vi "dashboard.vi"() -> ()   [LabVIEW 2022 SP3]
panel:
  in  "Stop":bool
  out "Write Count":i32
  out "Read Count":i32
  in  "Reset Communication":bool
  in  "USB Port":refnum<visa-resource-name>
  out "u":dbl format="%.2g"
  out "D":dbl format="%.2g"
  out "I":dbl format="%.2g"
  out "P":dbl format="%.2g"
  in  "Tau D (s)":dbl=11.370000000000003 min=0.0 max=30.0 step=0.01 format="%.2g"
  in  "Kd":dbl=46.0 min=0.0 max=50.0 step=0.01 format="%.2g"
  in  "Ki":dbl=49.920000000000016 min=0.0 max=50.0 step=0.01 format="%.2g"
  in  "Kp":dbl=37.15999999999997 min=0.0 max=50.0 step=0.01 format="%.2g"
  in  "Motor Enable":bool
  in  "Speed Reference (RPM)":dbl=100.0 min=0.0 max=1500.0 step=50.0 format="%#.3g"
  out "Flag AntiWindUp":bool
  in  "Tau Error (s)":dbl=8.649999999999995 min=0.0 max=30.0 step=0.01 format="%.2g"
  out "Filtered Error (°)":dbl
  out "Error (°)":dbl
  out "Controller":cluster{" P":dbl, "I":dbl, "D":dbl, "u":dbl}(graph)
  out "Error":cluster{" error":dbl, "Filtered_error":dbl}(graph)
  out "IR Sensors":bool[](array[boolean])
  in  "Right Motor Speed (RPM)":dbl(slide) min=-1500.0 max=1500.0 step=100.0 scale=-1500.0..1500.0
  in  "Left Motor Speed (RPM)":dbl(slide) min=-1500.0 max=1500.0 step=100.0 scale=-1500.0..1500.0
  in  "Manual Control":bool
  out "Left Motor":cluster{"l_sp":dbl, "l_speed":dbl}(graph)
  out "Right Motor":cluster{"r_sp":dbl, " r_speed":dbl}(graph)
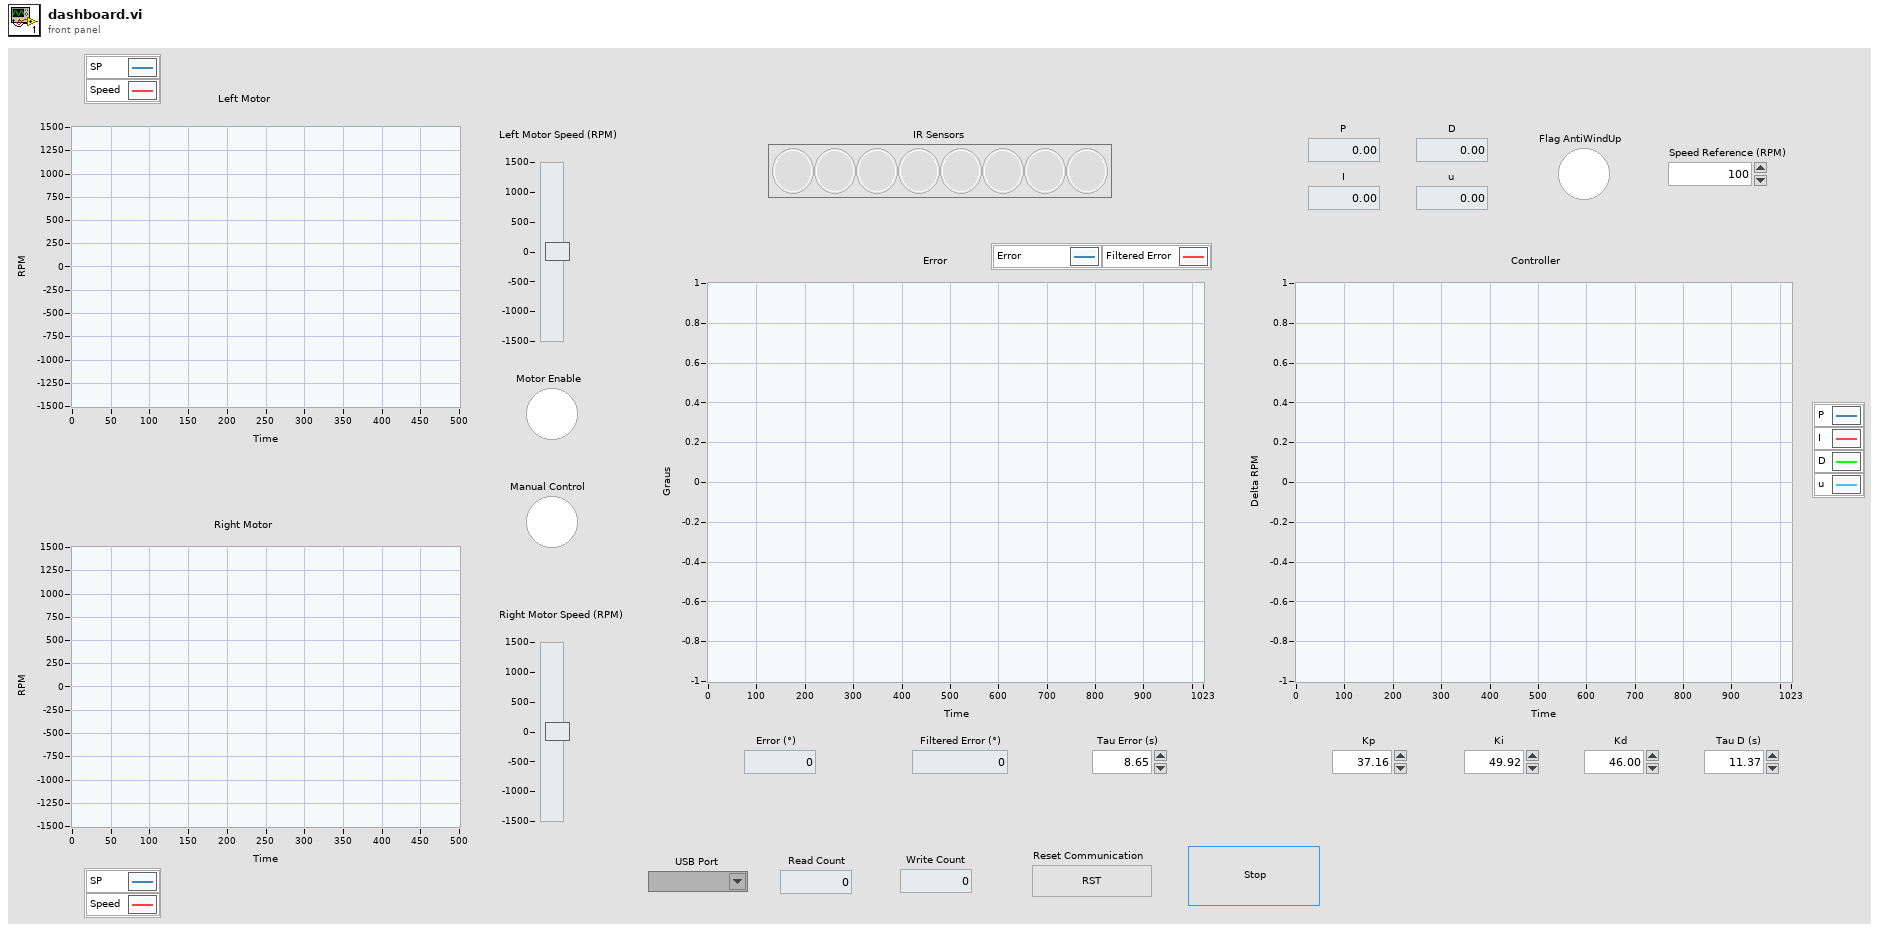
[diagram p1: front panel]
types:
  T1 = cluster{"Manual Control":bool, "Motor Enable":bool, "Left Motor Speed (RPM)":dbl, "Right Motor Speed (RPM)":dbl, "Tau Error (s)":dbl, "Kp":dbl, "Ki":dbl, "Kd":dbl, "Tau D (s)":dbl, "Speed Reference (RPM)":dbl, dbl, dbl, dbl, dbl, dbl, dbl}
  T2 = cluster{"l_sp":dbl, "l_speed":dbl, "r_sp":dbl, " r_speed":dbl, " error":dbl, "Filtered_error":dbl, " P":dbl, "I":dbl, "D":dbl, "u":dbl, "sat_flag":bool, " IR":bool[], "A_":dbl, " B_":dbl, " C_":dbl, "D_":dbl}
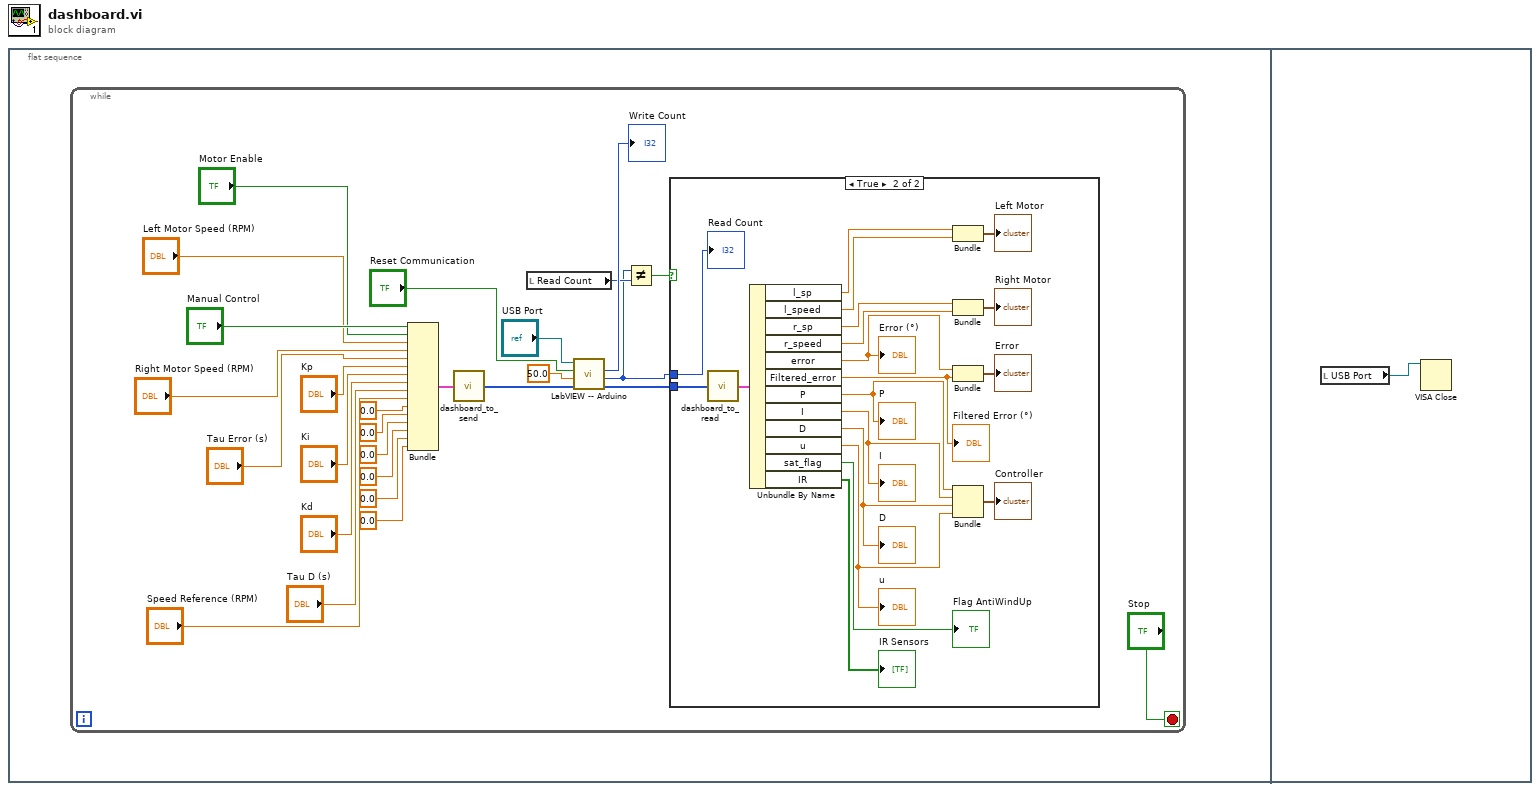
[diagram p0: block diagram]
diagram:
  n1 = flat-sequence {
    frame #0 {
      n2 = while {
        stop <- "Stop" stop-if-true
        n3 = Bundle("Manual Control"="Manual Control", "Motor Enable"="Motor Enable", "Left Motor Speed (RPM)"="Left Motor Speed (RPM)", "Right Motor Speed (RPM)"="Right Motor Speed (RPM)", "Tau Error (s)"="Tau Error (s)", "Kp"="Kp", "Ki"="Ki", "Kd"="Kd", "Tau D (s)"="Tau D (s)", "Speed Reference (RPM)"="Speed Reference (RPM)", 0.0, 0.0, 0.0, 0.0, 0.0, 0.0) -> (w6:T1)  [unwired: 1 in]
        n4 = call "dashboard_to_send.vi"("In"=w6) -> ("Output"=w5:u8[])
        n5 = local read "Read Count"() -> (w3:i32)
        n6 = call "LabVIEW -- Arduino.vi"("Data to Write"=w5, "Frequency Write"=50.0, "Reset"="Reset Communication", "VISA resource name"="USB Port") -> ("Read Data"=w1:u8[], "Read Count"=w2:i32, "Write Count"=→"Write Count":u16)  [unwired: 1 out]
        n7 = Not Equal?(x=w2, y=w3) -> (x != y?=w4:bool)
        n8 = case shown="True" w4 {
          tunnel: w2 -> [_ w46]
          tunnel: w1 -> [_ w45]
          frame False {
          }
          frame True {
            n9 = call "dashboard_to_read.vi"("In"=w45) -> ("Out"=w44:T2)
            n10 = Unbundle By Name(w44) -> ("l_sp"=w42:dbl, "l_speed"=w41:dbl, "r_sp"=w39:dbl, "r_speed"=w38:dbl, "error"=w33:dbl, "Filtered_error"=w32:dbl, "P"=w31:dbl, "I"=w30:dbl, "D"=w29:dbl, "u"=w28:dbl, "sat_flag"=→"Flag AntiWindUp":bool, "IR"=→"IR Sensors":bool[])
            "Error (°)" <- w33
            "Filtered Error (°)" <- w32
            "P" <- w31
            "I" <- w30
            "D" <- w29
            "u" <- w28
            n11 = Bundle("l_sp"=w42, "l_speed"=w41) -> (→"Left Motor":cluster{"l_sp":dbl, "l_speed":dbl})  [unwired: 1 in]
            n12 = Bundle("r_sp"=w39, "r_speed"=w38) -> (→"Right Motor":cluster{"r_sp":dbl, " r_speed":dbl})  [unwired: 1 in]
            n13 = Bundle("error"=w33, "Filtered_error"=w32) -> (→"Error":cluster{" error":dbl, "Filtered_error":dbl})  [unwired: 1 in]
            n14 = Bundle("P"=w31, "I"=w30, "D"=w29, "u"=w28) -> (→"Controller":cluster{" P":dbl, "I":dbl, "D":dbl, "u":dbl})  [unwired: 1 in]
            "Read Count" <- w46
          }
        }
      }
    }
    frame #1 {
      n15 = local read "USB Port"() -> (w47:refnum<visa-resource-name>)
      n16 = VISA Close(VISA resource name=w47) -> ()  [unwired: 1 in, 1 out]
    }
  }
